vi "Configure Attenuator.vi"(5 "Use Eletronic Attenuator (F)":bool, 7 "Auto Attenuator (T)":bool=TRUE, 8 "error in (no error)":errorcluster, 10 "Attenuator (dB)":u32, 11 "MXA in":refnum<class "MXA.lvclass">) -> (0 "error out":errorcluster, 3 "MXA out":refnum<class "MXA.lvclass">)   [LabVIEW 2020, in "MXA.lvclass"]
uses:
  MXA.lvclass
  C:/Sandbox/Git_Sandbox/WiSpry Test Framework source code (LV20)/WiSpry Test Framework/Instruments/Instrument.lvclass
  Instrument.lvclass/Instrument.ctl
  <instrlib>/Agilent MXA Series/Public/Configure/Configure Level (Normal).vi
  Instrument.lvclass
  <instrlib>/Agilent MXA Series/Agilent MXA Series.lvlib
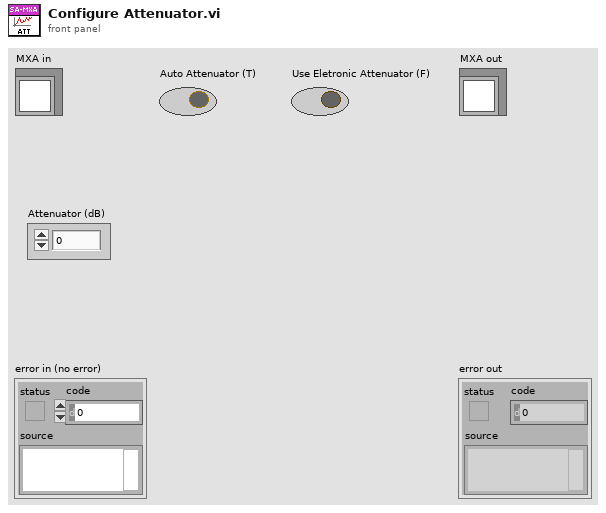
[diagram p1: front panel]
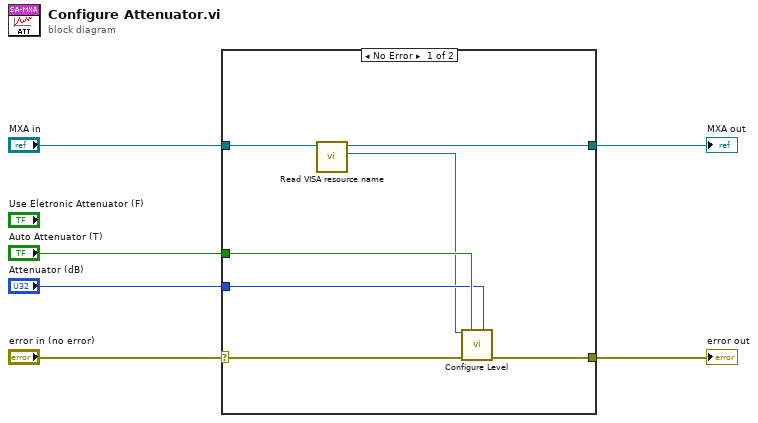
[diagram p0: block diagram]
diagram:
  n1 = case shown="No Error" "error in (no error)" {
    selector: "error in (no error)" -> [w10 w15]
    tunnel: "MXA in" -> [w13 w14]
    tunnel: [w9 w15] -> w6
    tunnel: [w12 w14] -> w5
    tunnel: "Auto Attenuator (T)" -> [w11 _]
    tunnel: "Attenuator (dB)" -> [w8 _]
    frame No Error {
      n2 = call "Read VISA resource name.vi"("Instrument in"=w13) -> ("VISA resource name"=w7:refnum<visa-resource-name>, "Instrument out"=w12:refnum<class "MXA.lvclass">)  [unwired: 9 in]
      n3 = call-poly <instrlib>:"Configure Level.vi"("VISA resource name"=w7, "Auto Mechanical Attenuation (T: Enable)"=w11, "Manual Mechanical Attenuation (10 dB)"=w8, "error in (no error)"=w10) -> ("error out"=w9:errorcluster)  [unwired: 10 in, 1 out]
    }
    frame Error {
    }
  }
  "error out" <- w6
  "MXA out" <- w5
